vi "Pre Launch Init.vi"(11 "DAQmx Actor in":refnum<class "DAQmx Actor.lvclass">) -> (0 "error out":errorcluster, 3 "DAQmx Actor out":refnum<class "DAQmx Actor.lvclass">)   [LabVIEW 2024, in "DAQmx Actor.lvlib" / "DAQmx Actor.lvclass"]
doc: "<p>(<strong>Filename</strong>: <span class=\"dnl\">Actor Framework.lvlib:Actor.lvclass:Pre Launch Init.vi</span>)</p>\n<p>Defines behavior that occurs after the <a href=\"nihelplauncher://docs/csh?context=lvcore_lvcomm_af_launch_nested_actor\">Launch Nested Actor</a> method is invoked but before the actor's Actor Core method begins running.</p>\n<p>By default, this method does nothing. A descendant class may override it to define behavior.</p>"
uses:
  DAQmx Actor.lvclass
  DAQmx Actor.lvclass/DAQmx Actor.ctl
  <vilib>/ActorFramework/Actor/Actor.lvclass
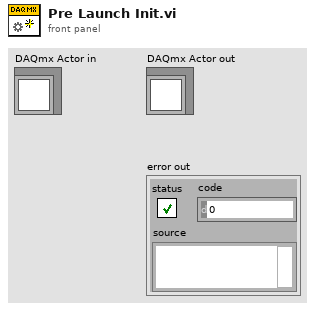
[diagram p1: front panel]
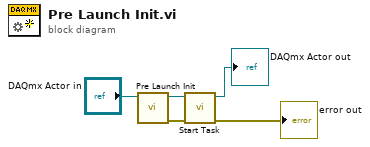
[diagram p0: block diagram]
diagram:
  n1 = call-parent "Pre Launch Init.vi"("Actor in"="DAQmx Actor in") -> ("error out"=w2:errorcluster, "Actor out"=w4:refnum<class "DAQmx Actor.lvclass">)  [unwired: 9 in]
  n2 = call "Start Task.vi"("error in (no error)"=w2, "DAQmx Actor in"=w4) -> ("error out"=→"error out":errorcluster, "DAQmx Actor out"=→"DAQmx Actor out":refnum<class "DAQmx Actor.lvclass">)  [unwired: 8 in]
